vi "All Check.vi"() -> ()   [LabVIEW 2018]
uses:
  CTL/Tags.ctl
panel:
  out "*(type *) &x":T1
  out "output array 2":string[](array[string])
  out "Array 5":string[](array[string])
  out "Array 4":u16[](array[numeric])
  out "array w/ subset deleted":string[](array[string])
  out "Array 3":T1[](array[typedef])
  out "size(s)":i32
  out "Array 2":string[](array[string])
  out "initialized array":string[][](array[string])
  in  "Stop":bool
  in  "Anchor Fore":bool
  in  "Mast Fore":bool
  in  "Manuvering Light":bool
  in  "Stern":bool
  in  "Mast Aft":bool
  in  "Anchor Aft":bool
  in  "Side Light  Port":bool
  in  "Side Light STBD":bool
  out "Array":string[](array[string])
  out "output array":string[][](array[string])
  in  "Power Supply":enum16{"2", "1"}(ring)
  in  "Lamp Selection":enum16{"1", "2"}(ring)
  in  "Lamp Selection Mode":enum16{"Manual", "Auto"}(ring)
  in  "Power Supply Mode":enum16{"Manual", "Auto"}(ring)
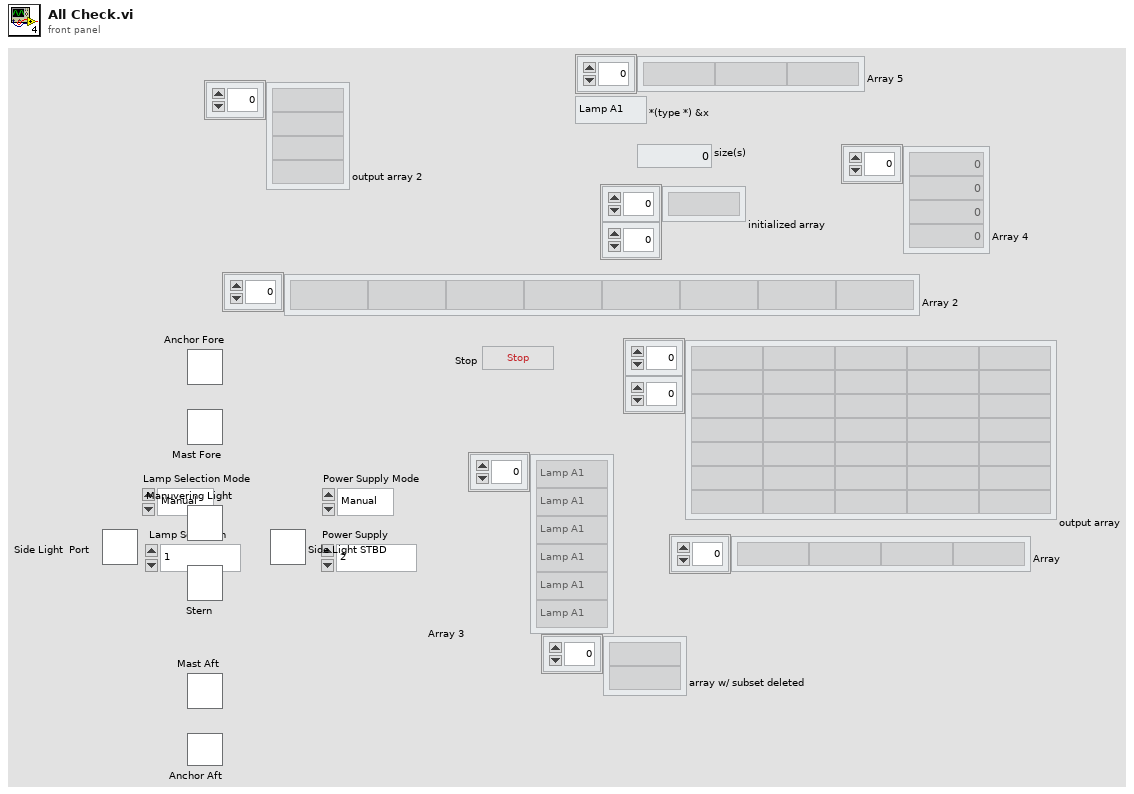
[diagram p1: front panel]
types:
  T1 = typedef "Tags.ctl" = enum16{"Lamp A1", "Lamp B1", "Lamp C1", "Lamp D1", "Lamp E1", "Lamp F1", "Lamp G1", "Lamp H1", "Lamp A2", "Lamp B2", "Lamp C2", "Lamp D2", "Lamp E2", "Lamp F2", "Lamp G2", "Lamp H2", "Ack A1", "Ack B1", "Ack C1", "Ack D1", "Ack E1", "Ack F1", "Ack G1", "Ack H1", "Ack A2", "Ack B2", "Ack C2", "Ack D2", "Ack E2", "Ack F2", "Ack G2", "Ack H2", "SSM", "SAS", "LSM", ""}
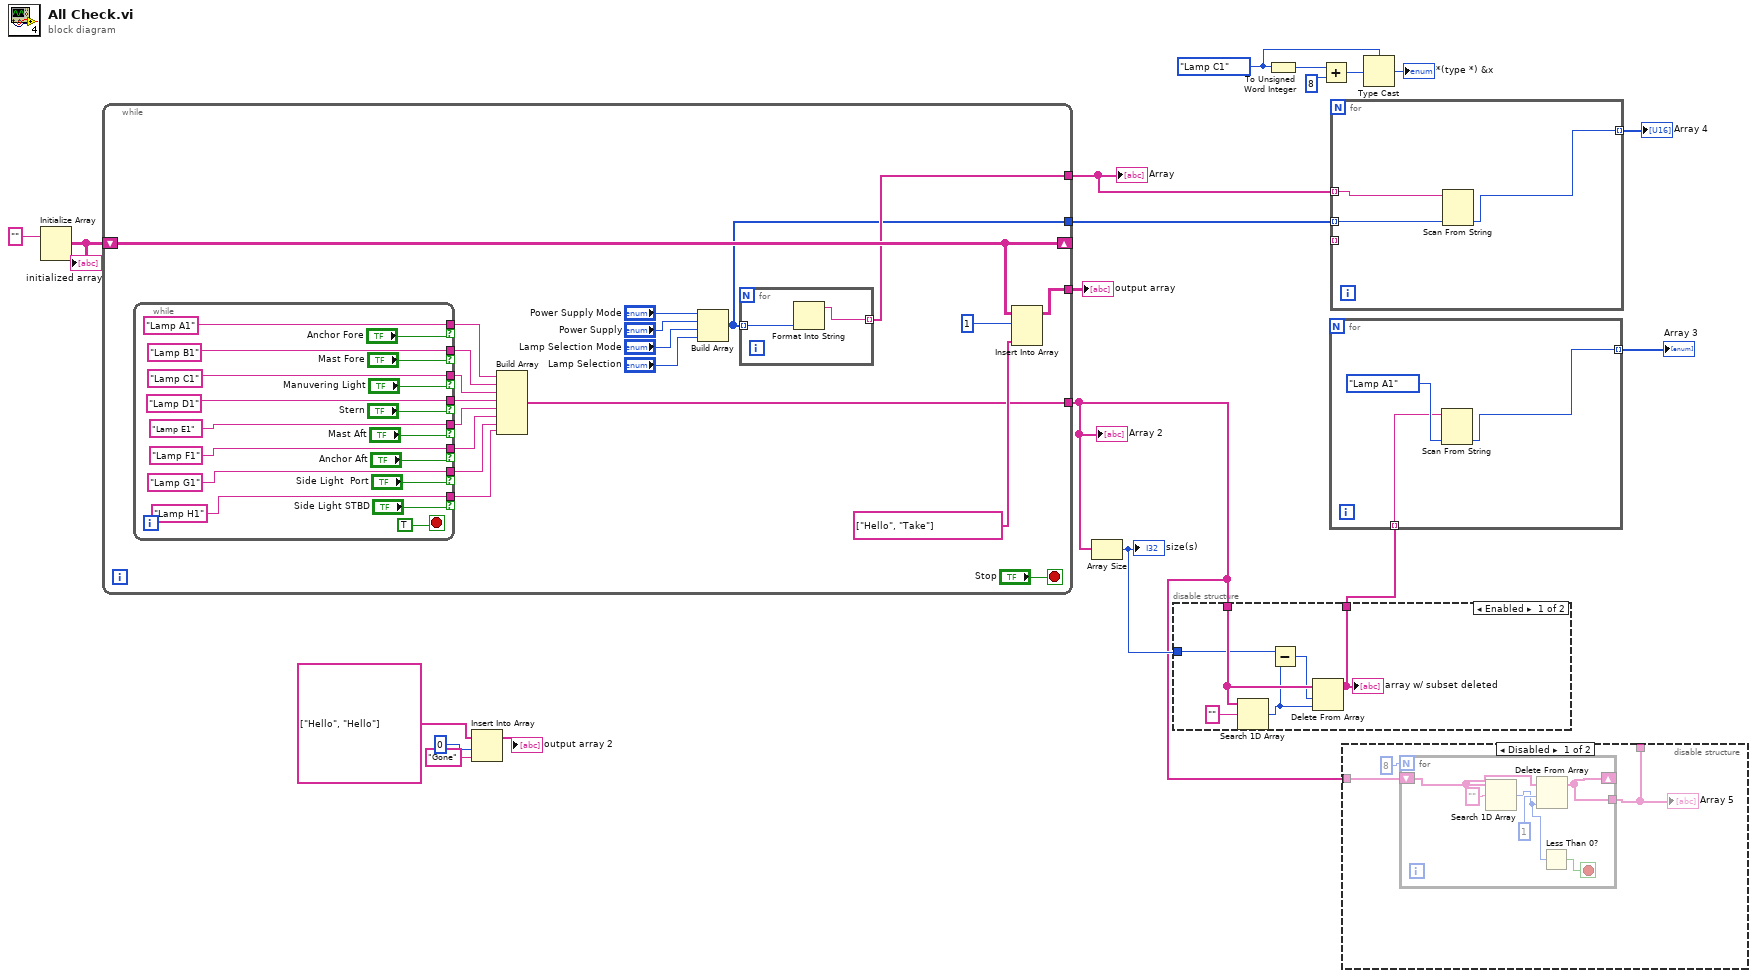
[diagram p0: block diagram]
diagram:
  w2 = Tags."Lamp C1" ("Tag")
  n1 = Initialize Array("") -> (w17:string[][])  [unwired: 2 in]
  "initialized array" <- w17
  n2 = while {
    tunnel: [w35] -> w19
    shift-right: [w26] -> _
    shift-left: w17 -> [w26]
    tunnel: [w23] -> w11
    tunnel: [w22] -> w14
    tunnel: [w20] -> w13
    stop <- "Stop" stop-if-true
    n3 = while {
      tunnel: ["Lamp A1"] -> w27 if="Anchor Fore"
      tunnel: ["Lamp B1"] -> w28 if="Mast Fore"
      tunnel: ["Lamp C1"] -> w29 if="Manuvering Light"
      tunnel: ["Lamp D1"] -> w30 if="Stern"
      tunnel: ["Lamp E1"] -> w31 if="Mast Aft"
      tunnel: ["Lamp F1"] -> w32 if="Anchor Aft"
      tunnel: ["Lamp G1"] -> w33 if="Side Light  Port"
      tunnel: ["Lamp H1"] -> w34 if="Side Light STBD"
      stop <- TRUE stop-if-true
    }
    n4 = Build Array(w27, w28, w29, w30, w31, w32, w33, w34) -> (w23:string[])
    n5 = Build Array("Power Supply Mode", "Power Supply", "Lamp Selection Mode", "Lamp Selection") -> (w20:u16[])
    n6 = for {
      tunnel: w20 -> [w58] mode=indexing
      tunnel: [w57] -> w22 mode=indexing
      n7 = Format Into String(w58) -> (resulting string=w57:string)  [unwired: 3 in, 1 out]
    }
    n8 = Insert Into Array(array=w26, index (row)=1, new element=string[] ["Hello", "Take"]) -> (w35:string[][])  [unwired: 1 in]
  }
  "output array" <- w19
  "Array 2" <- w11
  "Array" <- w14
  n9 = Insert Into Array(array=string[] ["Hello", "Hello"], index=0, new element="Gone" ("new element/subarray")) -> (→"output array 2":string[])
  n10 = Array Size(array=w11) -> (size(s)=w15:i32)
  "size(s)" <- w15
  n11 = disable-structure shown="Enabled" {
    disable-tunnel: w11 -> [w63 _]
    disable-tunnel: w15 -> [w62 _]
    disable-tunnel: [w59 _] -> w6
    frame Enabled {
      n12 = Search 1D Array(1D array=w63, element="") -> (index of element=w61:i32)  [unwired: 1 in]
      n13 = Subtract(x=w62, y=w61) -> (x-y=w60:i32)
      n14 = Delete From Array(array=w63, length=w60, index=w61) -> (array with subset deleted=w59:string[])  [unwired: 1 out]
      "array w/ subset deleted" <- w59
    }
    frame Disabled {
    }
  }
  n15 = To Unsigned Word Integer(number=w2) -> (unsigned 16bit integer=w3:u16)
  n16 = Add(x=w3, y=u16 8) -> (x+y=w5:u16)
  n17 = for {
    tunnel: [w67] -> w16 mode=indexing
    tunnel: w6 -> [w65] mode=indexing
    n18 = Scan From String(input string=w65, default 1=Tags."Lamp A1" ("Tag")) -> (output 1=w67:T1)  [unwired: 3 in, 3 out]
  }
  "Array 3" <- w16
  n19 = for {
    tunnel: [w69] -> _ mode=indexing
    tunnel: [w70] -> w12 mode=indexing
    tunnel: w14 -> [w69] mode=indexing
    tunnel: w13 -> [w68] mode=indexing
    n20 = Scan From String(input string=w69, default 1=w68) -> (output 1=w70:u16)  [unwired: 3 in, 3 out]
  }
  "Array 4" <- w12
  n21 = disable-structure shown="Disabled" {
    disable-tunnel: w11 -> [w72 _]
    disable-tunnel: [w71 _] -> _
    frame Disabled {
      n22 = for {
        N: 8 -> [_]
        shift-right: [w78] -> _
        shift-left: w72 -> [w79]
        tunnel: [w78] -> w71
        stop <- w74 stop-if-true
        n23 = Search 1D Array(1D array=w79, element="") -> (index of element=w75:i32)  [unwired: 1 in]
        n24 = Delete From Array(array=w79, length=1 ("index"), index=w75) -> (array with subset deleted=w78:string[])  [unwired: 1 out]
        n25 = Less Than 0?(x=w75) -> (x < 0?=w74:bool)
      }
      "Array 5" <- w71
    }
    frame Enabled {
    }
  }
  n26 = Type Cast(type=w2, x=w5) -> (*(type *) &x=→"*(type *) &x":T1)
